vi "Register VI(s).vi"   [LabVIEW 2020]
doc: "Register VI(s) to the localizer's registry. Automatically applies the current language to these VIs."
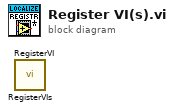
[diagram p0: block diagram]
diagram:
  n1 = call "RegisterVIs.vi"() -> ()  [unwired: 10 in, 2 out]
  n2 = call "RegisterVI.vi"() -> ()  [unwired: 10 in, 2 out]
